vi "Filter out owner.vi"(8 "error in":errorcluster, 9 "Include VI Lib?":bool, 10 "Owner":path, 11 "Linker.Read Info From File in":T2(array[cluster])) -> (0 "error out":errorcluster, 3 "Linker.Read Info From File out":T2(array[cluster]))   [LabVIEW 2020, in "SimpleDependencyInspector.lvlib"]
uses:
  SimpleDependencyInspector.lvlib
  <vilib>/Utility/lvfile.llb/LVFileType.ctl
  <vilib>/Utility/lvfile.llb/NI_FileType.lvlib
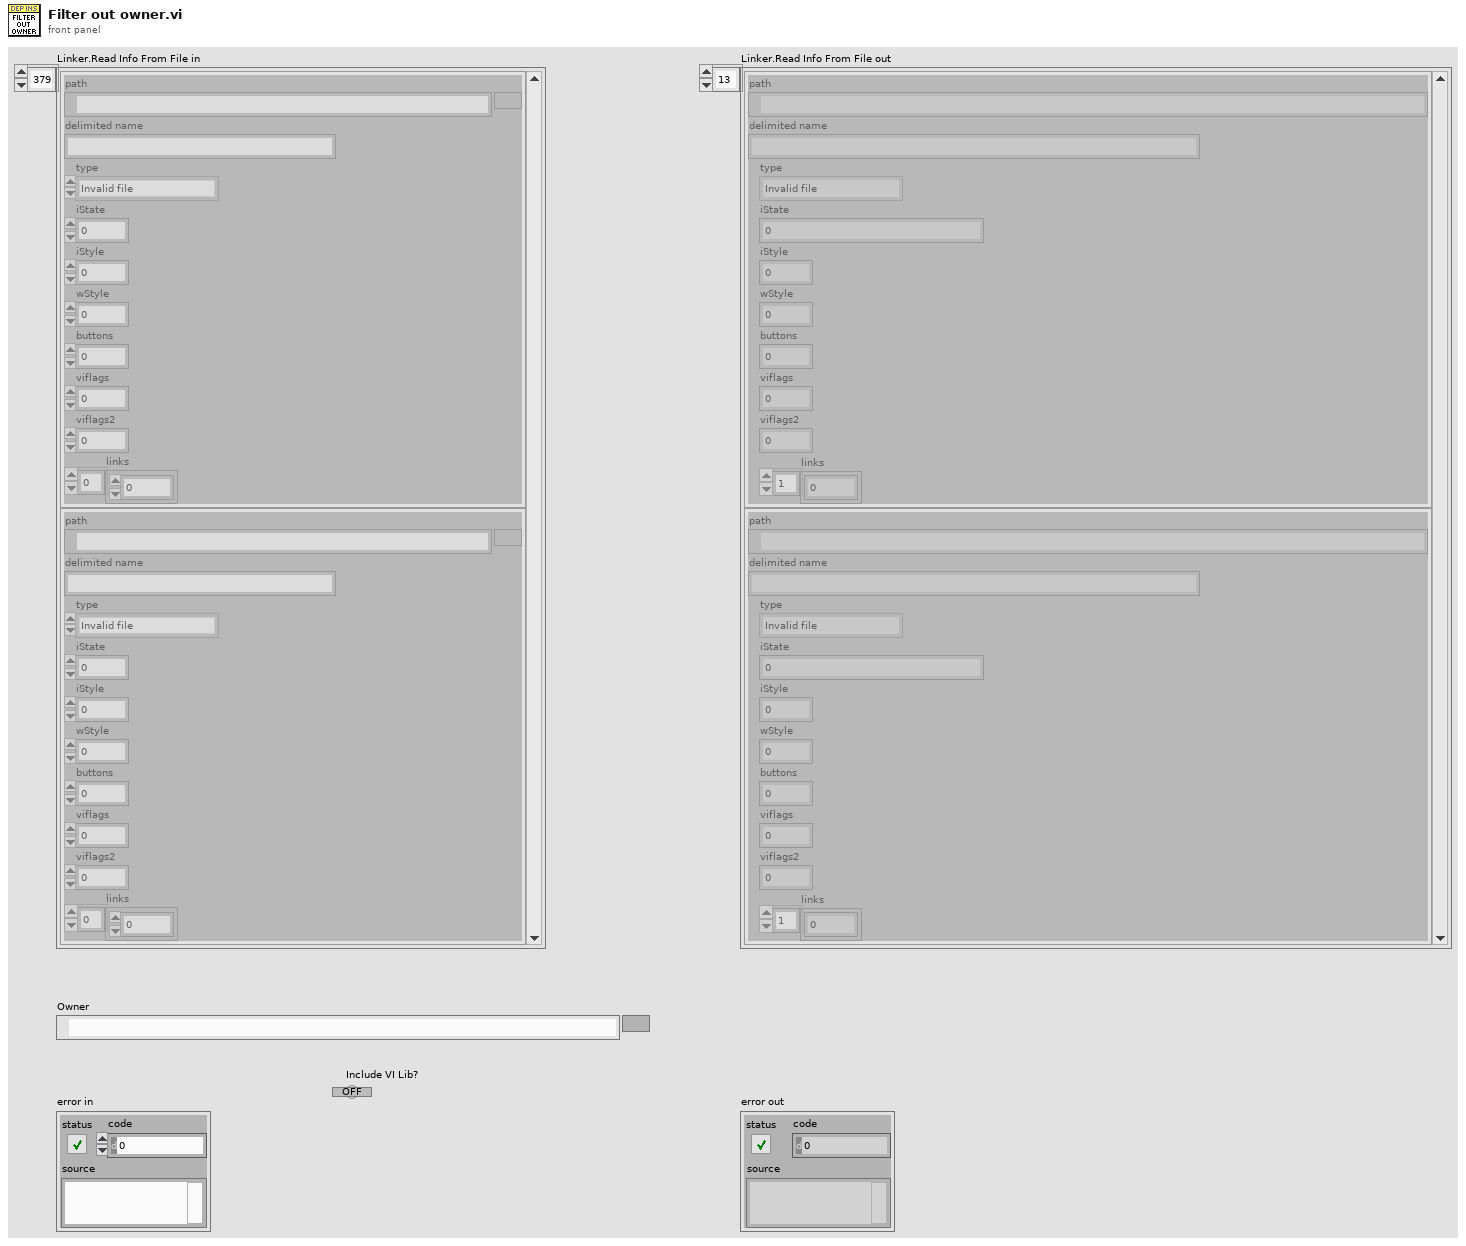
[diagram p1: front panel]
types:
  T1 = typedef "NI_FileType.lvlib/LVFileType.ctl" = enum32{"Invalid file", "Unknown type", "Instrument", "Control", "Polymorphic VI", "Project", "Library", "LVClass", "XControl", "XNode", "Shared library", ".NET assembly", "ActiveX interface", "CIN", "Run-time menu", "Palette menu", "Help file", "LLB", "XNode Edit Dependency", "Class Private Data Control", "Statechart", "MathScript .m file", "Ladder Diagram", "LVLibp", "XNode Build Dependency"}
  T2 = cluster{"path":path, "delimited name":string, "type":T1, "iState":u32, "iStyle":u16, "wStyle":u16, "buttons":u16, "viflags":u32, "viflags2":u32, "links":u32[]}[]
  T3 = cluster{"path":path, "delimited name":string, "type":T1, "iState":u32, "iStyle":u16, "wStyle":u16, "buttons":u16, "viflags":u32, "viflags2":u32, "links":u32[]}
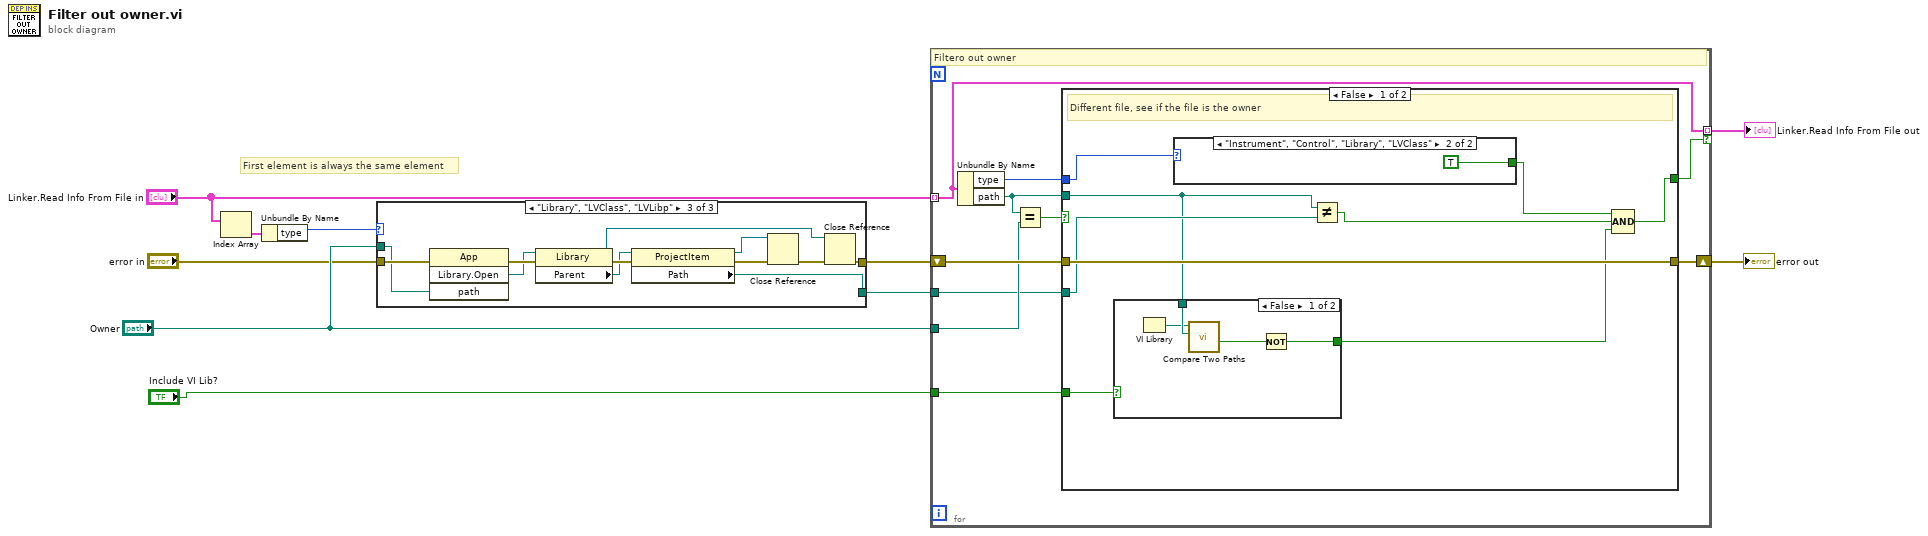
[diagram p0: block diagram]
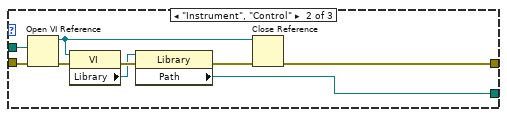
[diagram p3: hidden frame]
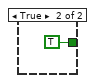
[diagram p4: hidden frame]
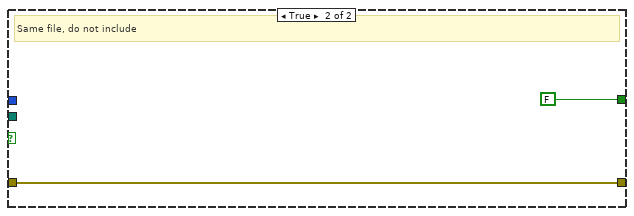
[diagram p6: hidden frame]
diagram:
  # "First element is always the same element"
  n1 = Index Array(array="Linker.Read Info From File in") -> (element=w8:T3)  [unwired: 1 in]
  n2 = Unbundle By Name(w8) -> ("type"=w7:T1)
  n3 = case shown="\"Library\", \"LVClass\", \"LVLibp\"" w7 {
    tunnel: "Owner" -> [_ w20 w30]
    tunnel: "error in" -> [w11 w19 w32]
    tunnel: [w11 w18 w22] -> w4
    tunnel: [_ w12 w25] -> w3
    frame Default {
    }
    frame "Instrument", "Control" {
      n4 = Open VI Reference(vi path=w20, error in (no error)=w19) -> (vi reference=w17:refnum<vi>, error out=w16:errorcluster)  [unwired: 4 in]
      n5 = property class="VI"(reference=w17, error in=w16) -> (error out=w15:errorcluster, "Library"=w13:refnum<vi>)  [unwired: 1 out]
      n6 = property class="Library"(reference=w13, error in=w15) -> (error out=w14:errorcluster, "Path"=w12:path)  [unwired: 1 out]
      n7 = Close Reference(reference=w17, error in (no error)=w14) -> (error out=w18:errorcluster)
    }
    frame "Library", "LVClass", "LVLibp" {
      n8 = invoke class="App" method="Library.Open"(error in=w32, "path"=w30) -> (error out=w31:errorcluster, "Open Library"=w28:refnum<vi>)  [unwired: 2 in, 2 out]
      n9 = property class="Library"(reference=w28, error in=w31) -> (reference out=w21:refnum<vi>, error out=w29:errorcluster, "Parent"=w26:refnum<vi>)
      n10 = property class="ProjectItem"(reference=w26, error in=w29) -> (reference out=w23:refnum<vi>, error out=w27:errorcluster, "Path"=w25:path)
      n11 = Close Reference(reference=w23, error in (no error)=w27) -> (error out=w24:errorcluster)
      n12 = Close Reference(reference=w21, error in (no error)=w24) -> (error out=w22:errorcluster)
    }
  }
  n13 = for {
    tunnel: "Linker.Read Info From File in" -> [w40] mode=indexing
    tunnel: "Owner" -> [w38]
    tunnel: [w40] -> w1 mode=indexing if=w36
    shift-right: [w41] -> w10
    shift-left: w4 -> [w42]
    tunnel: w3 -> [w35]
    tunnel: "Include VI Lib?" -> [w33]
    # "Filtero out owner"
    n14 = Unbundle By Name(w40) -> ("type"=w34:T1, "path"=w39:path)
    n15 = Equal?(x=w39, y=w38) -> (x = y?=w37:bool)
    n16 = case shown="False" w37 {
      tunnel: w39 -> [w45 _]
      tunnel: [w47 FALSE] -> w36
      tunnel: w42 -> [w51 w59]
      tunnel: [w51 w59] -> w41
      tunnel: w35 -> [w50 _]
      tunnel: w34 -> [w48 _]
      tunnel: w33 -> [w44 _]
      frame False {
        # "Different file, see if the file is the owner"
        n17 = case shown="False" w44 {
          tunnel: w45 -> [w55 _]
          tunnel: [w52 TRUE] -> w43
          frame False {
            n18 = VI Library() -> (path=w54:path)
            n19 = call <vilib>:"Compare Two Paths.vi"("Path 2"=w55, "Path 1"=w54) -> ("Path 2 Relative to Path 1?"=w53:bool)  [unwired: 6 in, 3 out]
            n20 = Not(x=w53) -> (.not. x?=w52:bool)
          }
          frame True {
          }
        }
        n21 = case shown="\"Instrument\", \"Control\", \"Library\", \"LVClass\"" w48 {
          tunnel: [_ TRUE] -> w46
          frame Default {
          }
          frame "Instrument", "Control", "Library", "LVClass" {
          }
        }
        n22 = Not Equal?(x=w45, y=w50) -> (x != y?=w49:bool)
        n23 = Compound Arithmetic op=AND(w46, w49, w43) -> (w47:bool)
      }
      frame True {
        # "Same file, do not include"
      }
    }
  }
  "Linker.Read Info From File out" <- w1
  "error out" <- w10
